vi "Enum Add.vi"(8 "error in (no error)":errorcluster, 10 "Typedef Enum Control Filepath (.ctl)":path, 11 "Item to Add":string) -> (0 "error out":errorcluster)   [LabVIEW 2014]
doc: "This VI will show you how to programmatically add elements to an enum or a ring.\nYou cannot run this code if the actual control is in memory. This means that you cannot change the control and use it at the same time."
panel:
  # "Overview: This VI will show you how to programmatically add elements to an enum or a ring.\nRequirements: LabVIEW 2012 (or compatible)\nInstructions:\n1. Open the enum or  ring control (.ctl) you want to add elements to (i.e. Enum Control.ctl) \n2. Specify the filepath of the control opened\n3. Run this VI and see the new elements in the opened control."
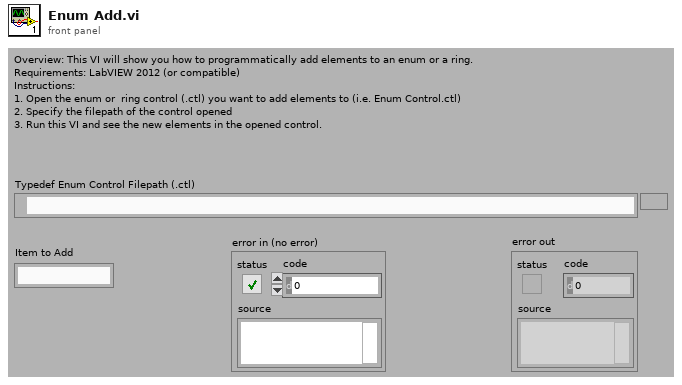
[diagram p1: front panel]
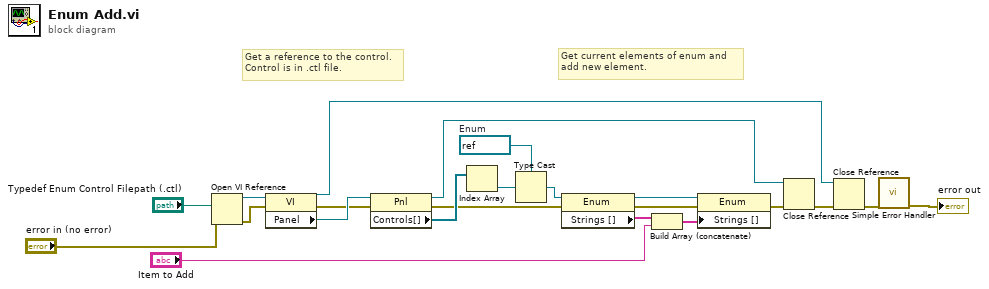
[diagram p0: block diagram]
diagram:
  w18 = refnum<vi> refnum  # Enum
  # "Get current elements of enum and\nadd new element."
  # "Get a reference to the control.\nControl is in .ctl file."
  n1 = Open VI Reference(vi path="Typedef Enum Control Filepath (.ctl)", error in (no error)="error in (no error)") -> (vi reference=w22:refnum<vi>, error out=w3:errorcluster)  [unwired: 4 in]
  n2 = property class="VI"(reference=w22, error in=w3) -> (reference out=w15:refnum<vi>, error out=w13:errorcluster, "Panel"=w21:refnum<vi>)
  n3 = property class="Pnl"(reference=w21, error in=w13) -> (reference out=w14:refnum<vi>, error out=w12:errorcluster, "Controls[]"=w20:refnum<vi>[])
  n4 = Index Array(array=w20) -> (element=w19:refnum<vi>)  [unwired: 1 in]
  n5 = Type Cast(type=w18, x=w19) -> (*(type *) &x=w4:refnum<vi>)
  n6 = property class="Enum"(reference=w4, error in=w12) -> (reference out=w10:refnum<vi>, error out=w7:errorcluster, "Strings []"=w9:string[])
  n7 = Build Array (concatenate)(w9, "Item to Add") -> (w8:string[])
  n8 = property class="Enum"(reference=w10, error in=w7, "Strings []"=w8) -> (error out=w6:errorcluster)  [unwired: 1 out]
  n9 = Close Reference(reference=w14, error in (no error)=w6) -> (error out=w11:errorcluster)
  n10 = Close Reference(reference=w15, error in (no error)=w11) -> (error out=w5:errorcluster)
  n11 = call <vilib>:"Simple Error Handler.vi"("error in (no error)"=w5) -> ("error out"=→"error out":errorcluster)  [unwired: 4 in, 4 out]
